vi "dAngle_To_Encoder.vi"(8 "Current Encoder Pos":dbl, 10 "Angle Change":dbl) -> (3 "New Encoder Pos":dbl)   [LabVIEW 2012]
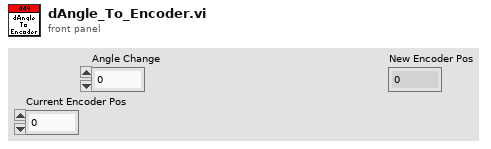
[diagram p1: front panel]
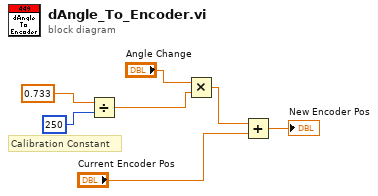
[diagram p0: block diagram]
diagram:
  # "Calibration Constant"
  n1 = Divide(x=0.733, y=250) -> (x/y=w3:dbl)
  n2 = Multiply(x="Angle Change", y=w3) -> (x*y=w6:dbl)
  n3 = Add(x=w6, y="Current Encoder Pos") -> (x+y=→"New Encoder Pos":dbl)
